vi "Update ID.vi"(10 "Entity ID":T1, 11 "Entity in":refnum<class "Entity.lvclass">) -> (3 "Entity out":refnum<class "Entity.lvclass">)   [LabVIEW 2020, in "Conditu2.lvlib" / "Entity.lvclass"]
uses:
  Entity.lvclass
  Entity ID.ctl
  Entity.lvclass/Entity.ctl
  Columns/ID/ID.lvclass/ID.ctl
  Columns/ID/ID.lvclass
  Conditu2.lvlib
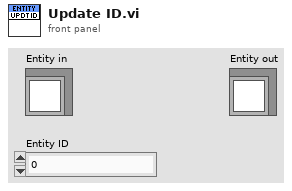
[diagram p1: front panel]
types:
  T1 = typedef "Conditu2.lvlib/Entity ID.ctl" = i64
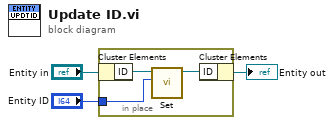
[diagram p0: block diagram]
diagram:
  n1 = in-place {
    in-place-border: "Entity ID" -> [w5]
    n2 = in-place-cluster #1("Entity in") -> ("ID"=w6:refnum<class "ID.lvclass">)
    n3 = call "Set.vi"("Entity ID"=w5, "ID in"=w6) -> ("ID out"=w4:refnum<class "ID.lvclass">)  [unwired: 9 in]
    n4 = in-place-cluster #1("ID"=w4) -> (→"Entity out":refnum<class "Entity.lvclass">)
  }
